vi "input_multichannel_producer.vi"(7 "Indices":i32[](array[numeric]), 8 "error in (no error)":errorcluster, 9 "aData Out":dbl[][](array[numeric]), 10 "Q":refnum<queue>) -> (0 "error out":errorcluster)   [LabVIEW 2025, in "LabJackEKG.lvlib"]
uses:
  LabJackEKG.lvlib
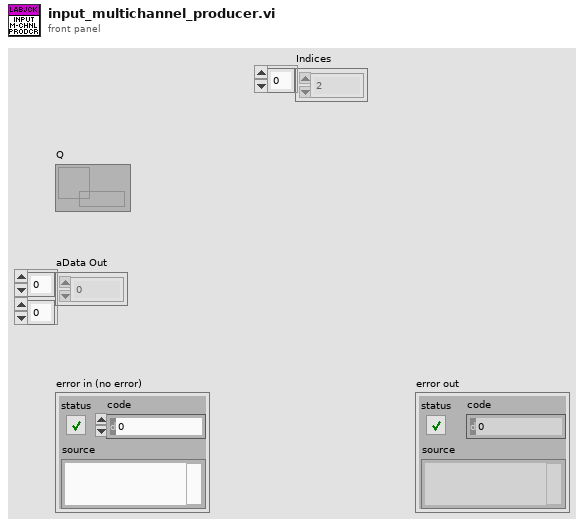
[diagram p1: front panel]
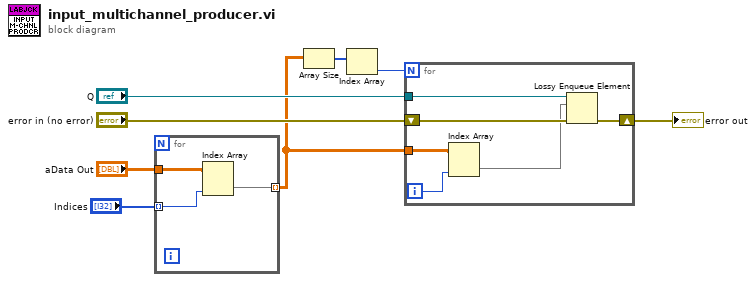
[diagram p0: block diagram]
diagram:
  n1 = for {
    tunnel: "Indices" -> [w11] mode=indexing
    tunnel: "aData Out" -> [w10]
    tunnel: [w9] -> w3 mode=indexing
    n2 = Index Array(array=w10, index (col)=w11) -> (element=w9:dbl[])  [unwired: 1 in]
  }
  n3 = Array Size(array=w3) -> (size(s)=w2:i32[])
  n4 = Index Array(array=w2) -> (element=w1:i32)  [unwired: 1 in]
  n5 = for {
    N: w1 -> [_]
    tunnel: "Q" -> [w17]
    shift-right: [w16] -> w8
    shift-left: "error in (no error)" -> [w15]
    tunnel: w3 -> [w14]
    i -> [w12]
    n6 = Index Array(array=w14, index (col)=w12) -> (element=w13:dbl[])  [unwired: 1 in]
    n7 = Lossy Enqueue Element(queue=w17, element=w13, error in (no error)=w15) -> (error out=w16:errorcluster)  [unwired: 3 out]
  }
  "error out" <- w8
